vi "charsequentialtstart.vi"() -> ()   [LabVIEW 2012]
uses:
  <vilib>/addons/Modulation/Digital/General/MT Generate PSK System Parameters(M).vi
  <instrlib>/niUSRP/niUSRP Write Tx Data (CDB Cluster).vi
  <vilib>/addons/Modulation/niDMT.lvlib
panel:
  in  "end of data?":bool
  out "error out 2":errorcluster
  out "String":string
  out "millisecond timer value":u32
  out "Entering into 2nd \n          Loop":string
  out "Symbol Rate\n[symbols/sec]":dbl=25000.0 format="%#.6p"
  in  "BPSK System Parameters 9":T1={"Samples per Symbol"=8, "symbol map"=[], "Differential PSK"=enum."disable", "PSK type"=0} caption="BPSK System Parameters" {"PSK type" items=["normal", "shifted", "offset"]; "symbol map" format="%.3f"}
  in  "BPSK System Parameters 8":T1={"Samples per Symbol"=8, "symbol map"=[], "Differential PSK"=enum."disable", "PSK type"=0} caption="BPSK System Parameters" {"PSK type" items=["normal", "shifted", "offset"]; "symbol map" format="%.3f"}
  in  "BPSK System Parameters 7":T1={"Samples per Symbol"=8, "symbol map"=[], "Differential PSK"=enum."disable", "PSK type"=0} caption="BPSK System Parameters" {"PSK type" items=["normal", "shifted", "offset"]; "symbol map" format="%.3f"}
  in  "BPSK System Parameters 6":T1={"Samples per Symbol"=8, "symbol map"=[], "Differential PSK"=enum."disable", "PSK type"=0} caption="BPSK System Parameters" {"PSK type" items=["normal", "shifted", "offset"]; "symbol map" format="%.3f"}
  in  "BPSK System Parameters 5":T1={"Samples per Symbol"=8, "symbol map"=[], "Differential PSK"=enum."disable", "PSK type"=0} caption="BPSK System Parameters" {"PSK type" items=["normal", "shifted", "offset"]; "symbol map" format="%.3f"}
  in  "BPSK System Parameters 4":T1={"Samples per Symbol"=8, "symbol map"=[], "Differential PSK"=enum."disable", "PSK type"=0} caption="BPSK System Parameters" {"PSK type" items=["normal", "shifted", "offset"]; "symbol map" format="%.3f"}
  in  "BPSK System Parameters 3":T1={"Samples per Symbol"=8, "symbol map"=[], "Differential PSK"=enum."disable", "PSK type"=0} caption="BPSK System Parameters" {"PSK type" items=["normal", "shifted", "offset"]; "symbol map" format="%.3f"}
  in  "Tab Control":T2(tab)
  in  "Enter control signal (1,2 or 3)":string
  in  "Packet Parameters":T3={"Guard Bits "=30, "Sync Bits"=20, "Message Bits"=128}
  in  "Packet Pad \n[samples]":i32=200
  in  "Blank Frame \n[samples]":i32=500
  out "Number of Packets in Message":i32=46
  in  "PN sequence order\nfor Sync Bits":i32=31 caption="PN sequence order (9)"
  in  "Packet Repeat":i32=2
  in  "Pulse Shaping Filter Parameters":T4={"Alpha"=0.5, "Filter Length"=6, "TX Filter"=enum."Root Raised Cos"} caption="Pulse Shaping Filter" {"Alpha" format="%.2f"}
  in  "Tx Parameters":T5={"Tx IQ Sampling\nRate [s/sec]"=500000.0, "Tx Frequency [Hz]"=2500000000.0, "Tx Gain [dB]"=0.0, "Tx Antenna"="TX1"} {"Tx Gain [dB]" format="%#.6p"; "Tx Frequency [Hz]" format="%#.6p"; "Tx IQ Sampling\nRate [s/sec]" format="%#.6p"}
  out "Actual Tx Parameters":T5={"Tx IQ Sampling\nRate [s/sec]"=200000.0, "Tx Frequency [Hz]"=2500000000.0, "Tx Gain [dB]"=0.0, "Tx Antenna"="TX1"} {"Tx Gain [dB]" format="%#.6p"; "Tx Frequency [Hz]" format="%#.6p"; "Tx IQ Sampling\nRate [s/sec]" format="%#.6p"}
  in  "USRP IP address":refnum<k15>="192.168.10.2"
  out "error out":errorcluster
  in  "Queue Length":i32=10
  out "Transmission\n       Stop":bool
  out "Constellation Graph":T6(graph)
  in  "autoscale":bool
  out "millisecond timer value 2":u32
  out "x = y?":bool
  out "Transmission\n      Time":bool
  out "Message Text 3":string="Two roads diverged in a yellow wood,\nAnd sorry I could not travel both\nAnd be one traveler, long I stood\nAnd looked down one as far as I could\nTo where it bent in the undergrowth.\n\nThen took the other, as just as fair,\nAnd having perhaps the better claim,\nBecause it was grassy and wanted wear;\nThough as for that the passing there\nHad worn them really about the same.\n\nAnd both that morning equally lay\nIn leaves no step had trodden black.\nOh, I kept the first for another day!\nYet knowing how way leads on to way,\nI doubted if I should ever come back.\n\nI shall be telling this with a sigh\nSomewhere ages and ages hence:\nTwo roads diverged in a wood, and I--\nI took the one less traveled by,\nAnd that has made all the difference.\n"
  out "M-PSK (4)":i32
  # "Guard\nBand"
  # "Sync\nSeq"
  # "Packet\nNumber"
  # "Pad\nData"
  # "Blank\nFrame"
  # "Data"
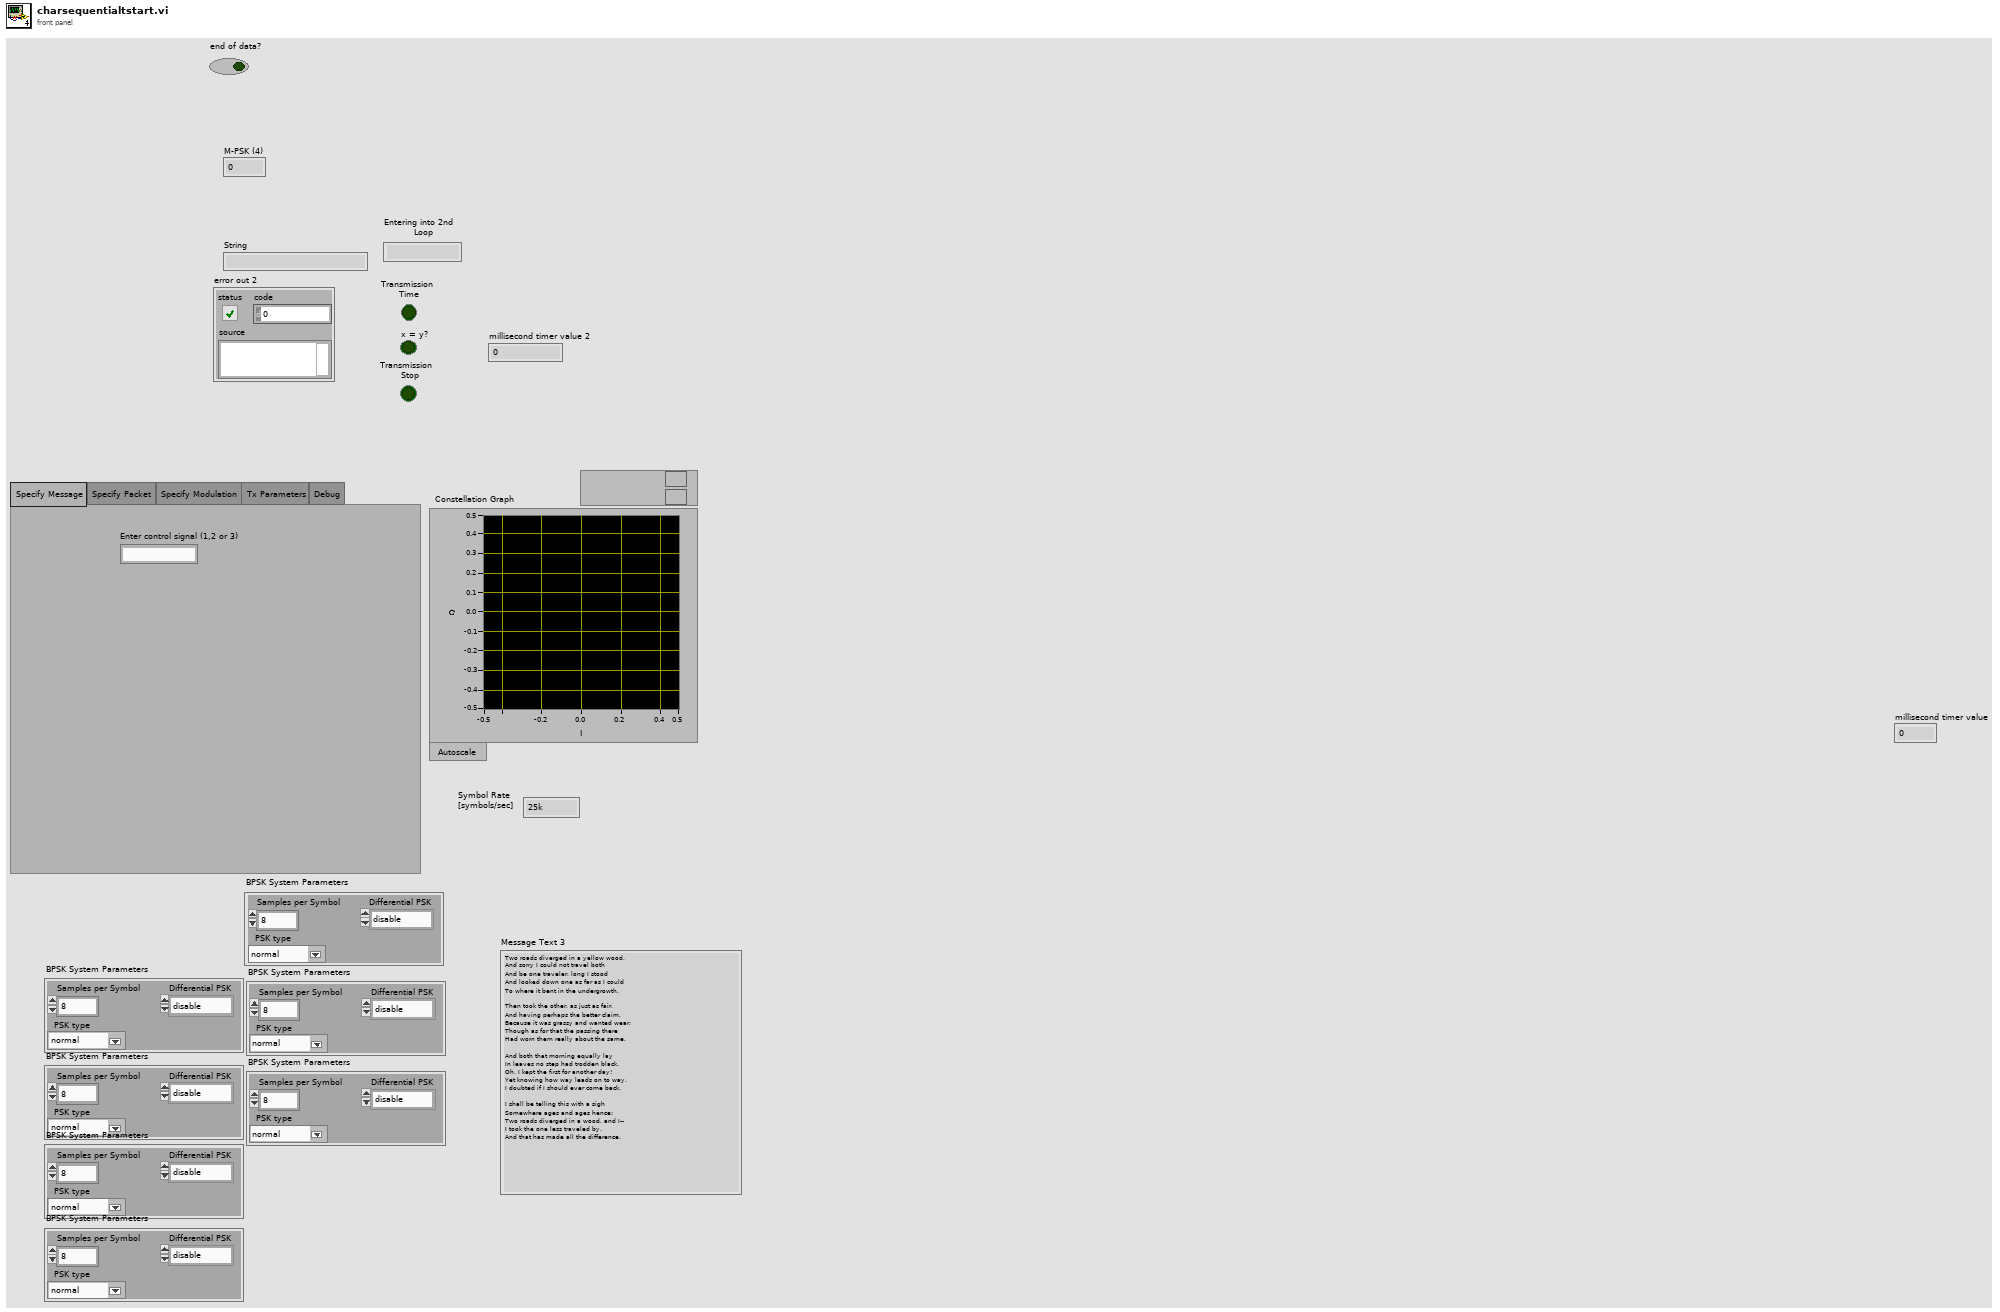
[diagram p1: front panel]
types:
  T1 = cluster{"Samples per Symbol":i32, "symbol map":cdb[], "Differential PSK":enum16{"disable", "enable"}, "PSK type":u16}
  T2 = enum32{"Specify Message", "Specify Packet", "Specify Modulation", "Tx Parameters", "Debug"}
  T3 = cluster{"Guard Bits ":i32, "Sync Bits":i32, "Message Bits":i32}
  T4 = cluster{"Alpha":dbl, "Filter Length":i32, "TX Filter":enum16{"none", "Raised Cosine", "Root Raised Cos", "Gaussian"}}
  T5 = cluster{"Tx IQ Sampling\nRate [s/sec]":dbl, "Tx Frequency [Hz]":dbl, "Tx Gain [dB]":dbl, "Tx Antenna":string}
  T6 = cluster{"Decimated Array":dbl[], "Decimated Array":dbl[]}[]
  T7 = cluster{"samples per symbol (16)":i32, "symbol map":cdb[], "differential PSK":enum16{"disable", "enable"}, "PSK type":u16}
  T8 = cluster{"s? t:f":cluster{"t0":dbl, "dt":dbl, "Y":cdb[]}, i32}
  T9 = cluster{"output complex waveform":cluster{"t0":dbl, "dt":dbl, "Y":cdb[]}, i32}
  T10 = cluster{"constellation":dbl[], "oversampled data":dbl[]}[]
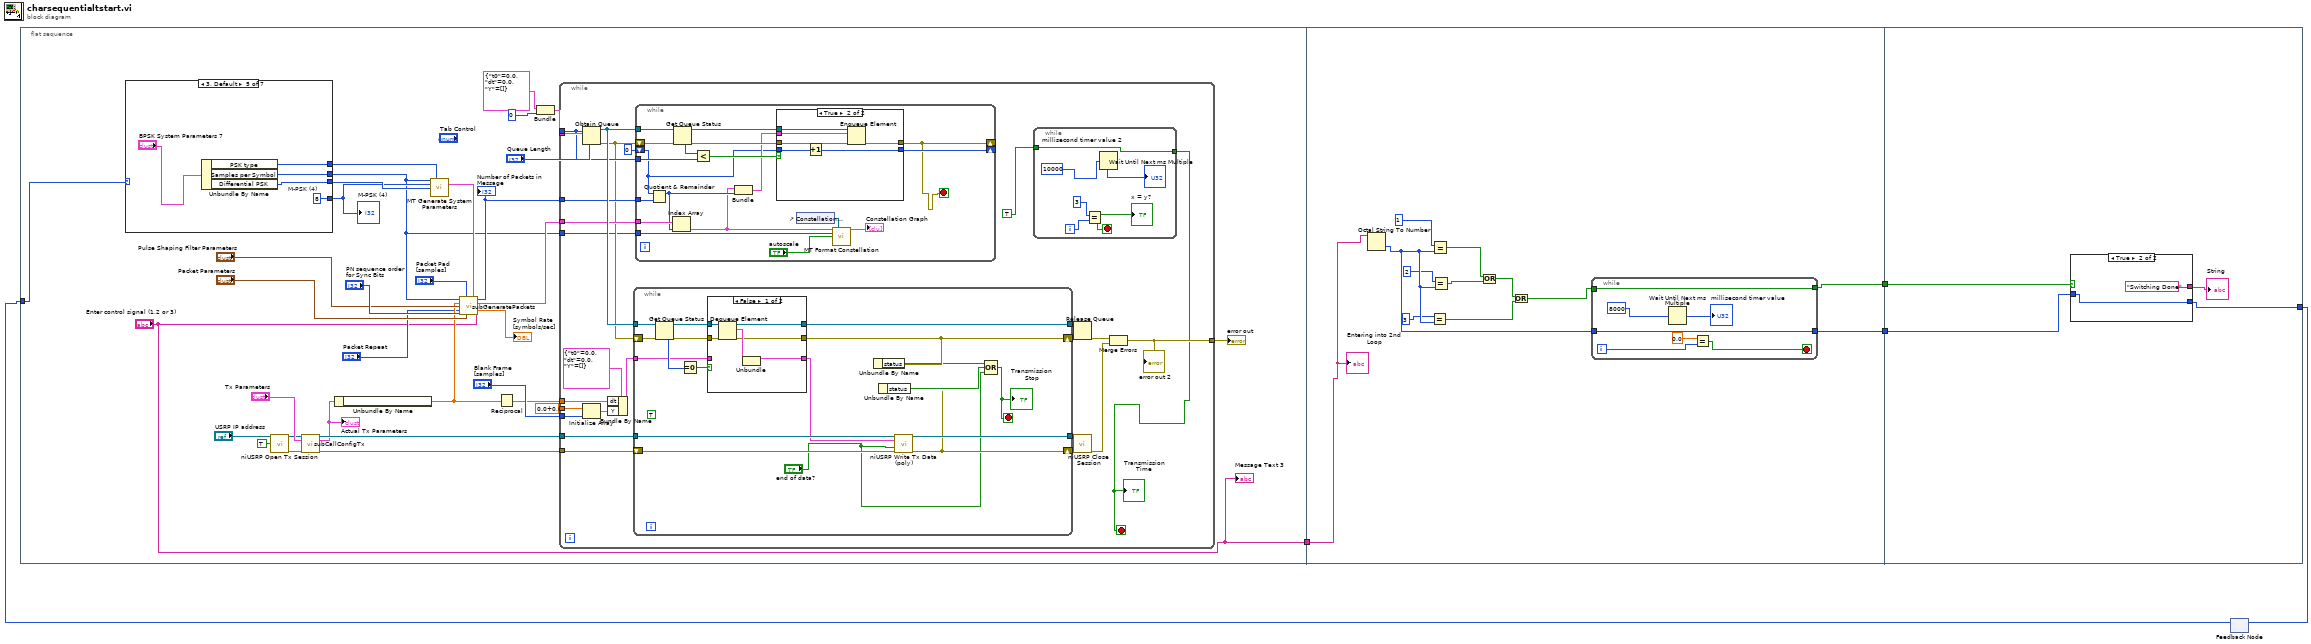
[diagram p0: block diagram]
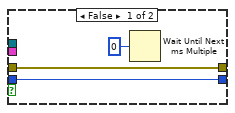
[diagram p2: hidden frame]
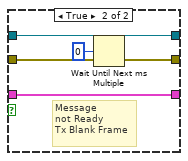
[diagram p3: hidden frame]
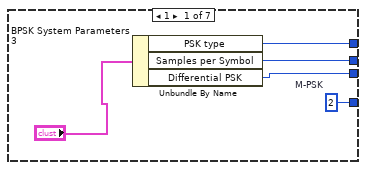
[diagram p4: hidden frame]
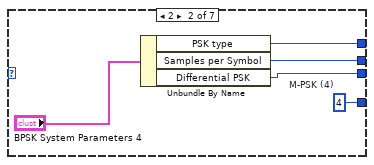
[diagram p5: hidden frame]
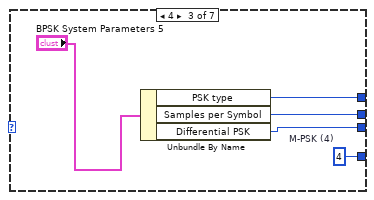
[diagram p6: hidden frame]
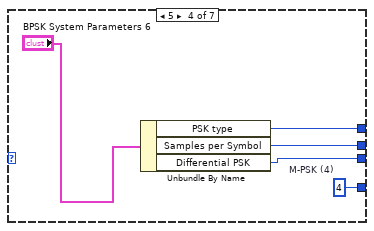
[diagram p7: hidden frame]
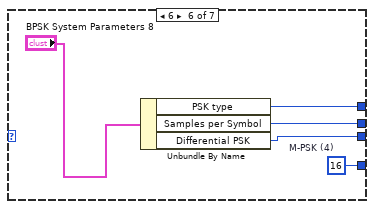
[diagram p8: hidden frame]
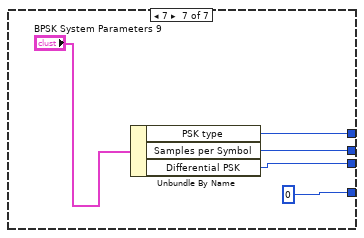
[diagram p9: hidden frame]
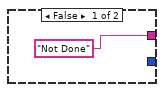
[diagram p10: hidden frame]
diagram:
  n1 = flat-sequence {
    tunnel: ["Enter control signal (1,2 or 3)"] -> w5
    tunnel: w1 -> [w7]
    tunnel: w5 -> [w160]
    tunnel: [w162] -> w4
    tunnel: [w161] -> w3
    tunnel: w4 -> [w181]
    tunnel: w3 -> [w180]
    tunnel: [w179] -> w2
    frame #0 {
      n2 = case shown="3, Default" w7 {
        tunnel: [w126 w131 w138 w143 w148 w154 w157] -> w10
        tunnel: [w127 w132 w137 w142 w147 w153 w158] -> w37
        tunnel: [w129 w134 w139 w144 w146 w152 0 ("M-PSK (4)")] -> w27
        tunnel: [w128 w133 w136 w141 w149 w151 w159] -> w16
        frame 1 {
          w129 = 2  # M-PSK
          n3 = Unbundle By Name("BPSK System Parameters 3") -> ("PSK type"=w128:u16, "Samples per Symbol"=w126:i32, "Differential PSK"=w127:enum16{"disable", "enable"})
        }
        frame 2 {
          w134 = 4  # M-PSK (4)
          n4 = Unbundle By Name("BPSK System Parameters 4") -> ("PSK type"=w133:u16, "Samples per Symbol"=w131:i32, "Differential PSK"=w132:enum16{"disable", "enable"})
        }
        frame 4 {
          w139 = 4  # M-PSK (4)
          n5 = Unbundle By Name("BPSK System Parameters 5") -> ("PSK type"=w136:u16, "Samples per Symbol"=w138:i32, "Differential PSK"=w137:enum16{"disable", "enable"})
        }
        frame 5 {
          w144 = 4  # M-PSK (4)
          n6 = Unbundle By Name("BPSK System Parameters 6") -> ("PSK type"=w141:u16, "Samples per Symbol"=w143:i32, "Differential PSK"=w142:enum16{"disable", "enable"})
        }
        frame 3, Default {
          w146 = 8  # M-PSK (4)
          n7 = Unbundle By Name("BPSK System Parameters 7") -> ("PSK type"=w149:u16, "Samples per Symbol"=w148:i32, "Differential PSK"=w147:enum16{"disable", "enable"})
        }
        frame 6 {
          w152 = 16  # M-PSK (4)
          n8 = Unbundle By Name("BPSK System Parameters 8") -> ("PSK type"=w151:u16, "Samples per Symbol"=w154:i32, "Differential PSK"=w153:enum16{"disable", "enable"})
        }
        frame 7 {
          n9 = Unbundle By Name("BPSK System Parameters 9") -> ("PSK type"=w159:u16, "Samples per Symbol"=w157:i32, "Differential PSK"=w158:enum16{"disable", "enable"})
        }
      }
      "M-PSK (4)" <- w27
      n10 = call <instrlib>:"niUSRP Open Tx Session.vi"("device names"="USRP IP address", "reset"=TRUE) -> ("session handle out"=w20:refnum<k15>, "error out"=w19:errorcluster)  [unwired: 12 in]
      n11 = call "subCallConfigTx.vi"("session handle"=w20, "Tx Parameters"="Tx Parameters", "error in"=w19) -> ("session handle out"=w26:refnum<k15>, "Actual Tx Parameters"=w25:T5, "error out"=w29:errorcluster)  [unwired: 10 in]
      "Actual Tx Parameters" <- w25
      n12 = Unbundle By Name(w25) -> ("Tx IQ Sampling\nRate [s/sec]"=w11:dbl)
      n13 = call-poly <vilib>:"MT Generate System Parameters.vi"("samples per symbol (16)"=w10, "PSK type"=w16, "M-PSK (4)"=w27, "differential PSK"=w37) -> ("PSK system parameters"=w17:T7)  [unwired: 9 in, 2 out]
      n14 = call "subGeneratePackets.vi"("Samples per Symbol"=w10, "Packet Pad \n[samples]"="Packet Pad \n[samples]", "PSK system parameters"=w17, "Tx IQ Sampling\nRate [s/sec]"=w11, "Pulse Shaping Filter Parameters"="Pulse Shaping Filter Parameters", "Packet Repeat"="Packet Repeat", "PN sequence order\nfor Sync Bits"="PN sequence order\nfor Sync Bits", "Packet Parameters"="Packet Parameters", "Message Text"="Enter control signal (1,2 or 3)") -> ("Number of Packets"=w24:i32, "Packets"=w31:cluster{"t0":dbl, "dt":dbl, "Y":cdb[]}[], "Symbol Rate"=→"Symbol Rate\n[symbols/sec]":dbl)  [unwired: 4 in]
      "Number of Packets in Message" <- w24
      n15 = Reciprocal(x=w11) -> (1/x=w28:dbl)
      n16 = Bundle("s? t:f"=cluster{"t0":dbl, "dt":dbl, "Y":cdb[]} {"t0"=0.0, "dt"=0.0, "Y"=[]}, 0) -> (w33:T8)  [unwired: 1 in]
      n17 = while {
        tunnel: cdb 0.0+0.0i ("element") -> [w62]
        tunnel: "Blank Frame \n[samples]" -> [w61]
        tunnel: w33 -> [w55]
        tunnel: "Queue Length" -> [w53]
        tunnel: w31 -> [w52]
        tunnel: w29 -> [w51]
        tunnel: w28 -> [w48]
        tunnel: w26 -> [w47]
        tunnel: w24 -> [w46]
        tunnel: [w41] -> w15
        tunnel: w10 -> [w40]
        stop <- w38 stop-if-true
        n18 = Obtain Queue(max queue size (-1, unlimited)=w53, element data type=w55) -> (queue out=w60:refnum<queue>, error out=w44:errorcluster)  [unwired: 3 in, 1 out]
        n19 = Initialize Array(w62, w61) -> (w59:cdb[])
        n20 = Bundle By Name(cluster=cluster{"t0":dbl, "dt":dbl, "Y":cdb[]} {"t0"=0.0, "dt"=0.0, "Y"=[]} ("s? t:f"), "dt"=w48, "Y"=w59) -> (w58:cluster{"t0":dbl, "dt":dbl, "Y":cdb[]})
        n21 = while {
          tunnel: w47 -> [w105]
          shift-right: [w102] -> w50
          shift-left: w51 -> [w106]
          tunnel: w60 -> [w114]
          tunnel: w58 -> [w111]
          tunnel: [w110] -> w57
          tunnel: [w104] -> w49
          shift-right: [w101] -> w56
          shift-left: w44 -> [w107]
          stop <- w98 stop-if-true
          (unwired) TRUE
          n22 = Get Queue Status(queue=w114, error in (no error)=w107) -> (queue out=w109:refnum<queue>, error out=w108:errorcluster, # elements in queue=w113:i32)  [unwired: 1 in, 5 out]
          n23 = Equal To 0?(x=w113) -> (x = 0?=w112:bool)
          n24 = case shown="False" w112 {
            tunnel: w111 -> [_ w124]
            tunnel: [w116 w124] -> w99
            tunnel: [w120 w122] -> w110
            tunnel: [w115 w123] -> w101
            tunnel: w109 -> [w119 w122]
            tunnel: w108 -> [w118 w123]
            frame False {
              n25 = Dequeue Element(queue=w119, error in (no error)=w118) -> (queue out=w120:refnum<queue>, element=w117:T8, error out=w115:errorcluster)  [unwired: 1 in, 1 out]
              n26 = Unbundle(w117) -> ("s? t:f"=w116:cluster{"t0":dbl, "dt":dbl, "Y":cdb[]})  [unwired: 1 out]
            }
            frame True {
              # "Message\nnot Ready\nTx Blank Frame"
              n27 = Wait Until Next ms Multiple(millisecond multiple=u32 0) -> ()  [unwired: 1 out]
            }
          }
          n28 = Unbundle By Name(w101) -> ("status"=w100:bool)
          n29 = call-poly <instrlib>:"niUSRP Write Tx Data (poly).vi"("session handle"=w105, "data"=w99, "end of data?"="end of data?", "error in (no error)"=w106) -> ("session handle out"=w104:refnum<k15>, "error out"=w102:errorcluster)  [unwired: 10 in]
          n30 = Unbundle By Name(w102) -> ("status"=w103:bool)
          n31 = Compound Arithmetic op=OR(w100, w103, "end of data?") -> (w98:bool)
          "Transmission\n       Stop" <- w98
        }
        n32 = while {
          tunnel: w60 -> [w87]
          shift-right: [w80] -> _
          shift-left: 0 -> [w76]
          tunnel: w52 -> [w77]
          tunnel: w53 -> [w79]
          tunnel: w46 -> [w78]
          shift-right: [w69] -> _
          shift-left: w44 -> [w82]
          tunnel: w40 -> [w72]
          stop <- w69 stop-if-true
          n33 = Quotient & Remainder(x=w76, y=w78) -> (x-y*floor(x/y)=w75:i32)  [unwired: 1 out]
          n34 = Index Array(array=w77, index=w75) -> (element=w70:cluster{"t0":dbl, "dt":dbl, "Y":cdb[]})
          n35 = Get Queue Status(queue=w87, error in (no error)=w82) -> (queue out=w86:refnum<queue>, error out=w83:errorcluster, # elements in queue=w85:i32)  [unwired: 1 in, 5 out]
          n36 = Less?(x=w85, y=w79) -> (x < y?=w84:bool)
          n37 = Bundle("output complex waveform"=w70, w75) -> (w81:T9)  [unwired: 1 in]
          n38 = case shown="True" w84 {
            tunnel: w83 -> [w88 w96]
            tunnel: w86 -> [_ w95]
            tunnel: [w88 w94] -> w69
            tunnel: w81 -> [_ w93]
            tunnel: w76 -> [w90 w92]
            tunnel: [w90 w91] -> w80
            frame False {
              n39 = Wait Until Next ms Multiple(millisecond multiple=u32 0) -> ()  [unwired: 1 out]
            }
            frame True {
              n40 = Increment(x=w92) -> (x+1=w91:i32)
              n41 = Enqueue Element(queue=w95, element=w93, error in (no error)=w96) -> (error out=w94:errorcluster)  [unwired: 1 in, 2 out]
            }
          }
          n42 = control-ref of="Constellation Graph"() -> (w73:refnum<vi>)
          n43 = call <vilib>:"MT Format Constellation.vi"("waveform"=w70, "constellation reference"=w73, "samples per symbol"=w72, "autoscale"="autoscale") -> ("constellation graph"=→"Constellation Graph":T10)  [unwired: 1 in, 10 out]
        }
        n44 = while {
          tunnel: TRUE -> [w68]
          tunnel: [w68] -> w38
          i -> [w66]
          stop <- w65 stop-if-true
          n45 = Equal?(x=3, y=w66) -> (x = y?=w65:bool)
          "x = y?" <- w65
          n46 = Wait Until Next ms Multiple(millisecond multiple=u32 10000) -> (millisecond timer value=→"millisecond timer value 2":u32)
        }
        "Transmission\n      Time" <- w38
        n47 = Release Queue(queue=w57, error in (no error)=w56) -> (error out=w43:errorcluster)  [unwired: 3 out]
        n48 = call <instrlib>:"niUSRP Close Session.vi"("session handle"=w49, "error in (no error)"=w50) -> ("error out"=w42:errorcluster)  [unwired: 13 in]
        n49 = Merge Errors(w43, w42) -> (w41:errorcluster)
        "error out 2" <- w41
      }
      "error out" <- w15
      "Message Text 3" <- "Enter control signal (1,2 or 3)"
    }
    frame #1 {
      n50 = Octal String To Number(4:w160) -> (0:w166:u32)  [unwired: 2 in, 1 out]
      n51 = Equal?(x=3, y=w166) -> (x = y?=w168:bool)
      n52 = Equal?(x=1, y=w166) -> (x = y?=w171:bool)
      n53 = Equal?(x=2, y=w166) -> (x = y?=w170:bool)
      n54 = Or(x=w171, y=w170) -> (x .or. y?=w169:bool)
      n55 = Or(x=w169, y=w168) -> (x .or. y?=w167:bool)
      n56 = while {
        tunnel: w167 -> [w177]
        tunnel: [w177] -> w162
        tunnel: w166 -> [w176]
        tunnel: [w176] -> w161
        i -> [w174]
        stop <- w173 stop-if-true
        n57 = Wait Until Next ms Multiple(millisecond multiple=u32 8000) -> (millisecond timer value=→"millisecond timer value":u32)
        n58 = Equal?(x=0.0, y=w174) -> (x = y?=w173:bool)
      }
      "Entering into 2nd \n          Loop" <- w160
    }
    frame #2 {
      n59 = case shown="True" w181 {
        tunnel: ["Not Done" "Switching Done"] -> w182
        tunnel: [_ w184] -> w179
        tunnel: w180 -> [_ w184]
        frame False {
        }
        frame True {
        }
      }
      "String" <- w182
    }
  }
  n60 = feedback #1() -> (w1:u32)  [unwired: 1 in]
  n61 = feedback-in #1(w2) -> ()
